vi "AE Camera Ball Image.vi"(7 "Update":bool, 10 "Camera Name":string, 11 "Fuel Image in":T1(plugin-control)) -> (3 "Fuel Image out":T1(plugin-control))   [LabVIEW 2025]
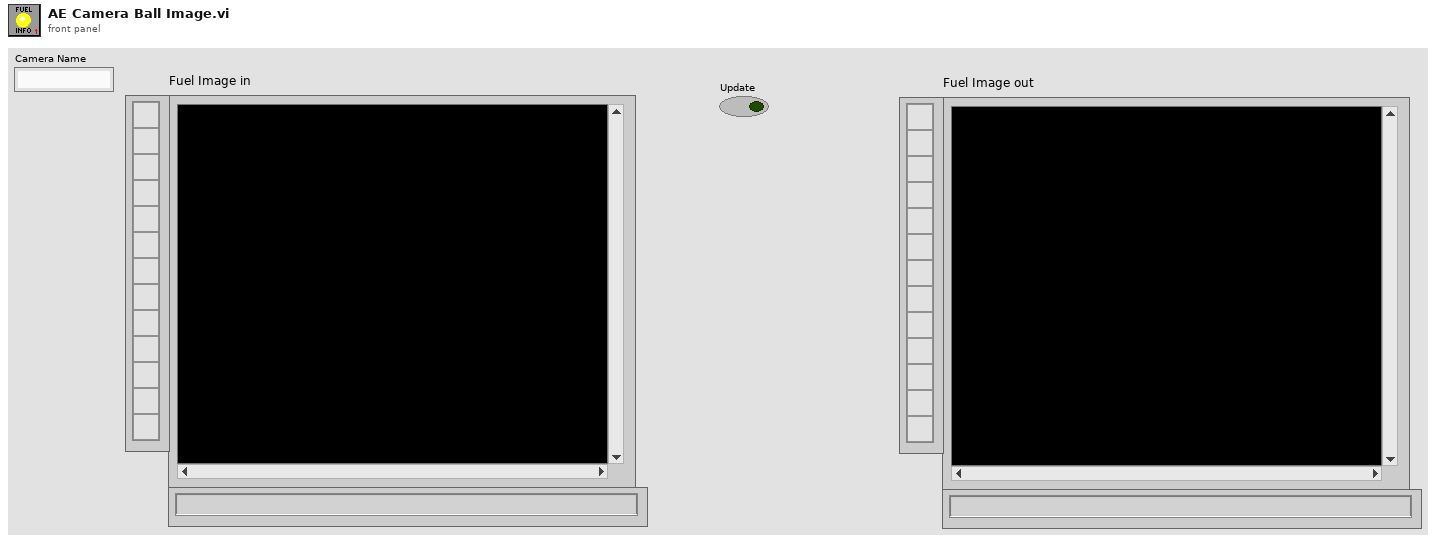
[diagram p1: front panel]
types:
  T1 = typedef "IMAQ Image.ctl" = refnum<image>
  T2 = typedef "Image Type" = u32
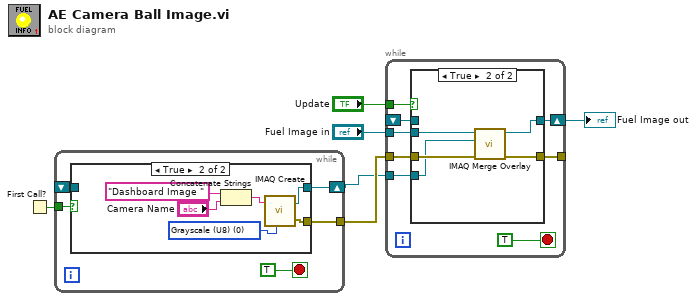
[diagram p0: block diagram]
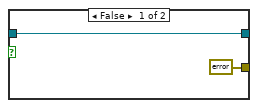
[diagram p2: hidden frame]
diagram:
  n1 = First Call?() -> (First Call?: T/F=w2:bool)
  n2 = while {
    tunnel: [w11] -> w3
    shift-right: [w7] -> w1
    shift-left: _ -> [w8]
    tunnel: w2 -> [w9]
    stop <- TRUE stop-if-true
    n3 = case shown="True" w9 {
      tunnel: [errorcluster {"status"=FALSE, "code"=0, "source"=""} ("error out") w17] -> w11
      tunnel: [w13 w16] -> w7
      tunnel: w8 -> [w13 _]
      frame False {
      }
      frame True {
        w18 = T2 0 items=["Grayscale (U8)", "Grayscale (I16)", "Grayscale (SGL)", "Complex (CSG)", "RGB (U32)", "HSL (U32)", "RGB (U64)", "Grayscale (U16)"] ("Image Type")
        n4 = Concatenate Strings("Dashboard Image " ("string"), "Camera Name") -> (w15:string)
        n5 = call "IMAQ Create"("Image Name"=w15, "Image Type"=w18) -> ("New Image"=w16:T1, "error out"=w17:errorcluster)  [unwired: 2 in, 1 out]
      }
    }
  }
  n6 = while {
    tunnel: "Update" -> [w27]
    tunnel: "Fuel Image in" -> [w26]
    shift-right: [w25] -> w4
    shift-left: _ -> [w24]
    tunnel: w3 -> [w22]
    tunnel: w1 -> [w21]
    tunnel: [w20] -> _
    stop <- TRUE stop-if-true
    n7 = case shown="True" w27 {
      tunnel: w26 -> [_ w34]
      tunnel: [w29 w31] -> w25
      tunnel: w24 -> [w29 _]
      tunnel: w22 -> [w28 w33]
      tunnel: w21 -> [_ w32]
      tunnel: [w28 w30] -> w20
      frame False {
      }
      frame True {
        n8 = call "IMAQ Merge Overlay"("error in (no error)"=w33, "Image Dst"=w32, "Image Src"=w34) -> ("error out"=w30:errorcluster, "Image Dst Out"=w31:T1)  [unwired: 7 in]
      }
    }
  }
  "Fuel Image out" <- w4
